vi "ZAlign.vi"(6 "Variant in":variant, 7 "Shift Pressed?":bool, 8 "error in (no error)":errorcluster, 10 "QD Combo Box Ref":refnum<vi>, 11 "QD Launch VI Ref":refnum<vi>) -> (0 "error out":errorcluster, 4 "Variant out":variant)   [LabVIEW 2014, in "ZAlign.lvlib"]
doc: "ZAlign.lvlib:ZAlign.vi\n----------------------------------------------\nQuickDrop Funktion ZAlign\n\nAuf einem Frontpanel werden alle Controls automatisch angeordnet und die Fenstergrösse eingestellt. Lokale nicht angeschlossene Controls werden unter Locals aufgeführt.\n\nTastenbefehl die ZAlign Funktion:\n1) CTRL-Space (QuickDrop starten)\n2) CTRL-A ZAlign ausführen\n\nCodebeschreibung:\n1) Das VI Fenster wird hier entsprechend der berechneten Werte eingestellt.\n2) Alle Controls erden an die neue Position verschoben.\n3) Zeichnen der Dekoartionsrahmen um die Controls\n\nDamit die Codestabilität hochgehalten werden kann, sind die VIs Passwortgeschützt. Bei Interesse und entsprechender Anfrage können die VIs aber auch entsperrt werden. \n\nInputs:\n---------------------\n- Variant in : LvVariant; \n- Shift Pressed? : Boolean; \n- error in (no error) : Cluster; \n- QD Combo Box Ref : Refnum; \n- QD Launch VI Ref : Refnum; \n\nOutputs:\n---------------------\n- error out : Cluster; \n- Variant out : LvVariant; \n\n----------------------------------------------\n16/03/2015\nZühlke Engineering AG\nCH-8952 Schlieren\nwww.zuehlke.com\n\nPLUGIN_DESCRIPTION: Zuehlke Quick Drop: ZAlign / 16.03.2015 \nPLUGIN_DEFAULT_SHORTCUT: A\n(Replace the \"$\" above with the character you wish to assign as the default shortcut for this plugin)."
uses:
  ZAlign/ZAlign.lvlib
panel:
  in  "Undo Name":string="Quick Drop Keyboard Shortcut"
  # "ZAlign!"
  # "Do not change the connector pane of this VI.\n\nSee the block diagram for directions on how to use this template."
  # "Specify the name of the Undo transaction"
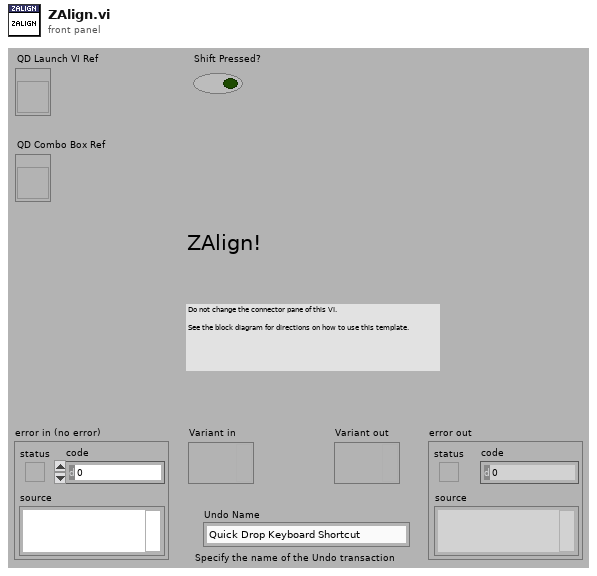
[diagram p1: front panel]
types:
  T1 = typedef "LVRectTypeDef.ctl" = cluster{"Left":i16, "Top":i16, "Right":i16, "Bottom":i16}
  T2 = cluster{"left":i16, "top":i16, "right":i16, "bottom":i16}
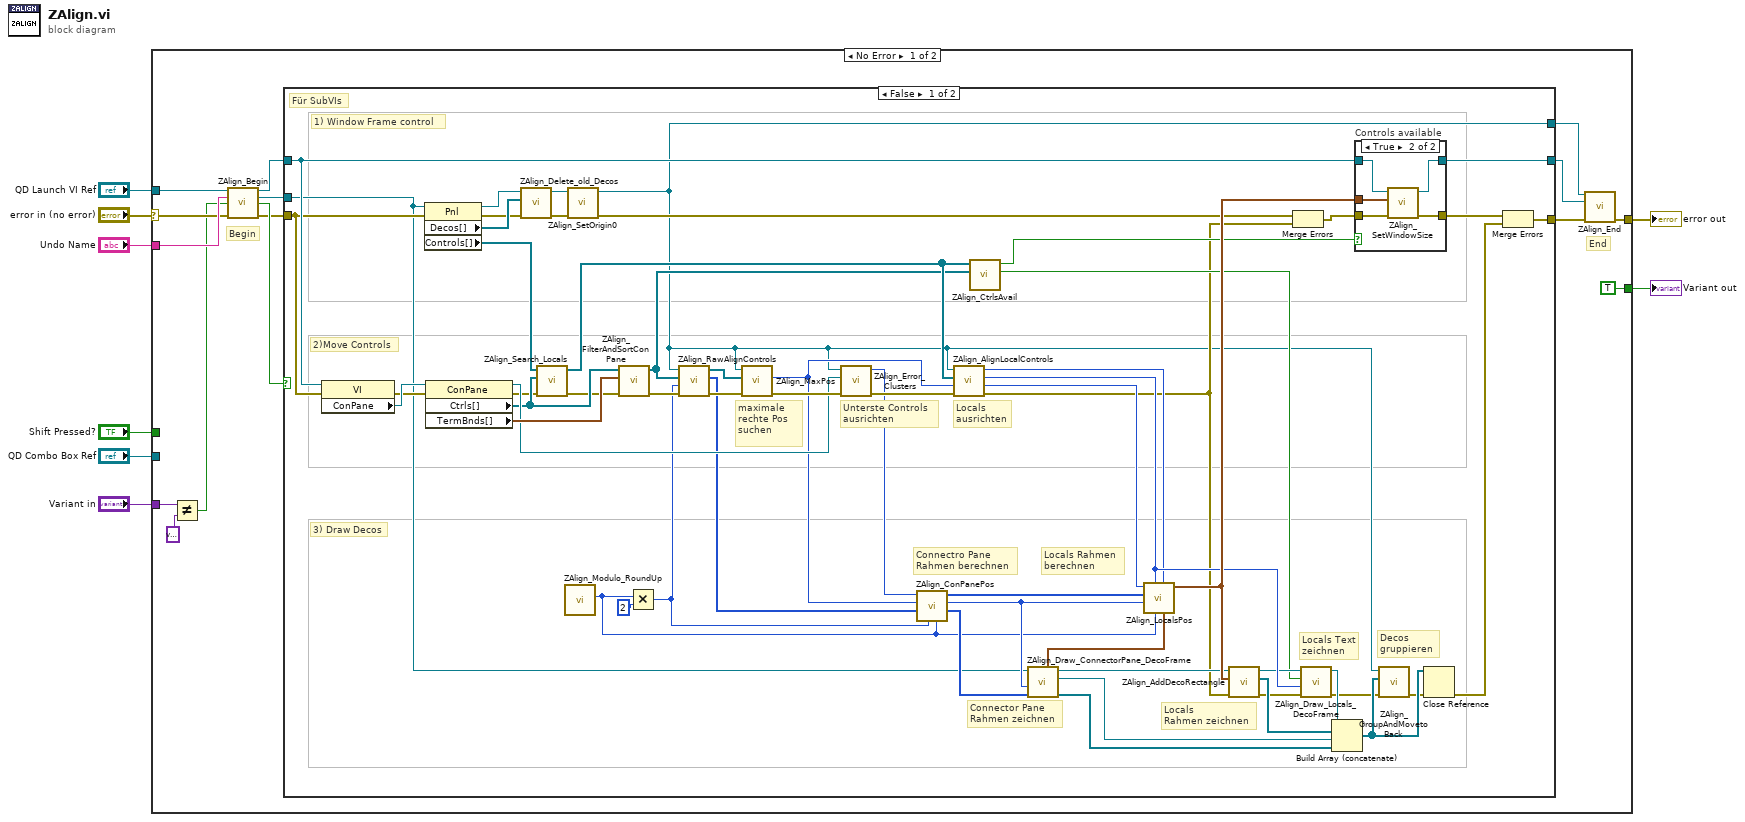
[diagram p0: block diagram]
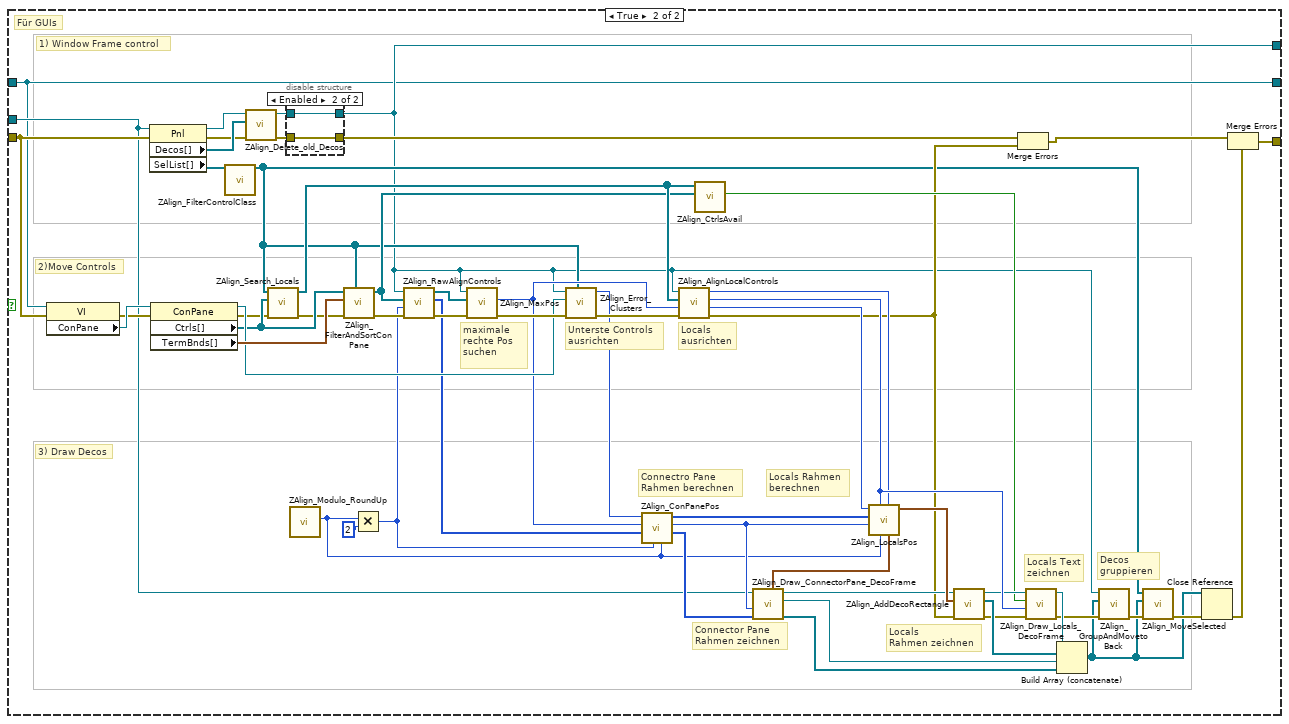
[diagram p3: hidden frame]
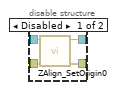
[diagram p4: hidden frame]
diagram:
  n1 = case shown="No Error" "error in (no error)" {
    selector: "error in (no error)" -> [w18 w150]
    tunnel: [w21 w150] -> w7
    tunnel: "QD Launch VI Ref" -> [w20 _]
    tunnel: "Shift Pressed?" -> [_ _]
    tunnel: "QD Combo Box Ref" -> [_ _]
    tunnel: "Variant in" -> [w11 _]
    tunnel: "Undo Name" -> [w23 _]
    tunnel: [TRUE _] -> w2
    frame No Error {
      # "End"
      # "Begin"
      n2 = Not Equal?(x=w11, y=variant) -> (x != y?=w9:bool)
      n3 = call "ZAlign_Begin.vi"("VI in"=w20, "Undo Name"=w23, "WithUndo"=w9, "error in (no error)"=w18) -> ("VIRef"=w16:refnum<vi>, "PanelRef"=w15:refnum<vi>, "SelectedElements?"=w19:bool, "error out"=w17:errorcluster)  [unwired: 8 in]
      n4 = case shown="False" w19 {
        tunnel: w17 -> [w26 w91]
        tunnel: [w65 w129] -> w14
        tunnel: w16 -> [w27 w88]
        tunnel: [w61 w88] -> w12
        tunnel: w15 -> [w25 w90]
        tunnel: [w24 w89] -> w13
        frame False {
          # "Für SubVIs"
          # "Locals Rahmen \nberechnen"
          # "Connectro Pane\nRahmen berechnen"
          # "3) Draw Decos"
          # "2)Move Controls"
          # "1) Window Frame control"
          # "Decos\ngruppieren"
          # "Locals Text\nzeichnen"
          # "Connector Pane\nRahmen zeichnen"
          # "Locals \nRahmen zeichnen"
          # "Locals\nausrichten"
          # "Unterste Controls \nausrichten"
          # "maximale\nrechte Pos\nsuchen"
          n5 = property class="VI"(reference=w27, error in=w26) -> (error out=w74:errorcluster, "ConPane"=w79:refnum<vi>)  [unwired: 1 out]
          n6 = property class="Pnl"(reference=w25, error in=w26) -> (reference out=w37:refnum<vi>, error out=w54:errorcluster, "Decos[]"=w67:refnum<vi>[], "Controls[]"=w35:refnum<vi>[])
          n7 = property class="ConPane"(reference=w79, error in=w74) -> (reference out=w75:refnum<vi>, error out=w38:errorcluster, "Ctrls[]"=w62:refnum<vi>[], "TermBnds[]"=w80:T1[])
          n8 = call "ZAlign_Delete_old_Decos.vi"("error in (no error)"=w54, "Decos[]"=w67, "Panel in"=w37) -> ("error out"=w51:errorcluster, "Panel out"=w36:refnum<vi>)  [unwired: 7 in]
          n9 = call "ZAlign_Search_Locals.vi"("error in (no error)"=w38, "Ctrls[]"=w62, "Controls[]"=w35) -> ("error out"=w52:errorcluster, "Array"=w71:refnum<vi>[])  [unwired: 7 in]
          n10 = call "ZAlign_Modulo_RoundUp.vi"() -> ("Grid_Size"=w31:i32)  [unwired: 10 in, 1 out]
          n11 = call "ZAlign_SetOrigin0.vi"("error in (no error)"=w51, "Panel in"=w36) -> ("error out"=w30:errorcluster, "reference out"=w24:refnum<vi>)  [unwired: 8 in]
          n12 = call "ZAlign_FilterAndSortConPane.vi"("error in (no error)"=w52, "TermBnds[]"=w80, "Ctrls[]"=w62) -> ("error out"=w76:errorcluster, "Ctrls[]out"=w50:refnum<vi>[])  [unwired: 7 in]
          n13 = Multiply(x=w31, y=i16 2) -> (x*y=w59:i32)
          n14 = call "ZAlign_RawAlignControls.vi"("error in (no error)"=w76, "Offset (Left and right)"=w59, "Refs"=w50, "Panel in"=w24) -> ("error out"=w77:errorcluster, "Positions"=w41:u32[], "Refs_Out"=w73:refnum<vi>[])  [unwired: 5 in]
          n15 = call "ZAlign_MaxPos.vi"("error in (no error)"=w77, "Objects"=w73, "Panel"=w24) -> ("error out"=w78:errorcluster, "Max right location"=w43:u32)  [unwired: 6 in, 1 out]
          n16 = call "ZAlign_Error_Clusters.vi"("Error in"=w78, "ConPane"=w75, "Panel"=w24) -> ("Error out"=w72:errorcluster, "Height"=w64:u32)  [unwired: 6 in, 1 out]
          n17 = call "ZAlign_ConPanePos.vi"("Grid_Size"=w31, "ScaledGridSize"=w59, "Positions"=w41, "Max right location"=w43, "Height"=w64) -> ("Positions-Grid"=w47:u32[], "Height+Grid"=w68:u32, "Positions+Grid+MaxRight"=w42:u32[])  [unwired: 4 in]
          n18 = call "ZAlign_AlignLocalControls.vi"("error in (no error)"=w72, "Max right location"=w43, "CtrlRefs"=w71, "Panel in"=w24) -> ("error out"=w28:errorcluster, "Bottom"=w40:u32, "Left"=w58:u32, "Max Right"=w44:u32)  [unwired: 4 in]
          n19 = call "ZAlign_CtrlsAvail.vi"("ConectedRefs"=w50, "LocalRefs"=w71) -> ("ConRefsAvail"=w49:bool, "RefsAvail"=w48:bool)  [unwired: 8 in]
          n20 = call "ZAlign_Draw_ConnectorPane_DecoFrame.vi"("RightPos"=w47, "Bottom"=w68, "Panel in"=w25) -> ("Deco refs"=w57:refnum<vi>[], "Decoration out"=w34:refnum<vi>, "owner refnumout"=w33:refnum<vi>, "rect"=w32:T2)  [unwired: 5 in]
          n21 = call "ZAlign_LocalsPos.vi"("rect in"=w32, "Max Right"=w44, "Grid_Size"=w31, "Left"=w58, "Height+Grid"=w68, "Positions+Grid+MaxRight"=w42, "Bottom"=w40) -> ("rect out"=w63:T2)  [unwired: 4 in]
          n22 = call "ZAlign_AddDecoRectangle.vi"("error in (no error)"=w28, "rect"=w63, "owner refnum"=w33) -> ("error out"=w53:errorcluster, "Decoration refnums"=w69:refnum<vi>[], "owner refnumout"=w56:refnum<vi>)  [unwired: 6 in]
          n23 = Merge Errors(w30, w28) -> (w29:errorcluster)
          n24 = call "ZAlign_Draw_Locals_DecoFrame.vi"("error in (no error)"=w53, "Left"=w58, "ControlsAvailable"=w49, "Generic in"=w56) -> ("error out"=w46:errorcluster, "Decoration out"=w70:refnum<vi>)  [unwired: 6 in]
          n25 = Build Array (concatenate)(w70, w69, w34, w57) -> (w66:refnum<vi>[])
          n26 = case "Controls available" shown="True" w48 {
            tunnel: w63 -> [_ w87]
            tunnel: [w81 w86] -> w61
            tunnel: [w82 w85] -> w55
            tunnel: w27 -> [w81 w84]
            tunnel: w29 -> [w82 w83]
            frame False {
            }
            frame True {
              n27 = call "ZAlign_SetWindowSize.vi"("error in (no error)"=w83, "rect"=w87, "VI in"=w84) -> ("error out"=w85:errorcluster, "reference out"=w86:refnum<vi>)  [unwired: 7 in]
            }
          }
          n28 = call "ZAlign_GroupAndMovetoBack.vi"("error in (no error)"=w46, "CtrlRefs"=w66, "Panel"=w24) -> ("error out"=w45:errorcluster)  [unwired: 8 in]
          n29 = Close Reference ("Close Ref")(reference=w66, error in (no error)=w45) -> (error out=w39:errorcluster)
          n30 = Merge Errors(w55, w39) -> (w65:errorcluster)
        }
        frame True {
          # "Für GUIs"
          # "Locals Rahmen \nberechnen"
          # "Connectro Pane\nRahmen berechnen"
          # "3) Draw Decos"
          # "2)Move Controls"
          # "1) Window Frame control"
          # "Decos\ngruppieren"
          # "Locals Text\nzeichnen"
          # "Connector Pane\nRahmen zeichnen"
          # "Locals \nRahmen zeichnen"
          # "Locals\nausrichten"
          # "Unterste Controls \nausrichten"
          # "maximale\nrechte Pos\nsuchen"
          n31 = property class="VI"(reference=w88, error in=w91) -> (error out=w137:errorcluster, "ConPane"=w142:refnum<vi>)  [unwired: 1 out]
          n32 = property class="Pnl"(reference=w90, error in=w91) -> (reference out=w107:refnum<vi>, error out=w121:errorcluster, "Decos[]"=w130:refnum<vi>[], "SelList[]"=w101:refnum<vi>[])
          n33 = property class="ConPane"(reference=w142, error in=w137) -> (reference out=w138:refnum<vi>, error out=w108:errorcluster, "Ctrls[]"=w126:refnum<vi>[], "TermBnds[]"=w143:T1[])
          n34 = call "ZAlign_FilterControlClass.vi"("SelList[]"=w101) -> ("CtrlRefArray"=w92:refnum<vi>[])  [unwired: 14 in]
          n35 = call "ZAlign_Delete_old_Decos.vi"("error in (no error)"=w121, "Decos[]"=w130, "Panel in"=w107) -> ("error out"=w94:errorcluster, "Panel out"=w95:refnum<vi>)  [unwired: 7 in]
          n36 = call "ZAlign_Search_Locals.vi"("error in (no error)"=w108, "Ctrls[]"=w126, "Controls[]"=w92) -> ("error out"=w119:errorcluster, "Array"=w134:refnum<vi>[])  [unwired: 7 in]
          n37 = disable-structure shown="Enabled" {
            disable-tunnel: w95 -> [w147 w149]
            disable-tunnel: [w146 w149] -> w89
            disable-tunnel: w94 -> [w145 w148]
            disable-tunnel: [w144 w148] -> w93
            frame Disabled {
              n38 = call "ZAlign_SetOrigin0.vi"("error in (no error)"=w145, "Panel in"=w147) -> ("error out"=w144:errorcluster, "reference out"=w146:refnum<vi>)  [unwired: 8 in]
            }
            frame Enabled {
            }
          }
          n39 = call "ZAlign_Modulo_RoundUp.vi"() -> ("Grid_Size"=w103:i32)  [unwired: 10 in, 1 out]
          n40 = call "ZAlign_FilterAndSortConPane.vi"("FilterCtrls[]"=w92, "error in (no error)"=w119, "TermBnds[]"=w143, "Ctrls[]"=w126) -> ("error out"=w139:errorcluster, "Ctrls[]out"=w118:refnum<vi>[])  [unwired: 6 in]
          n41 = Multiply(x=w103, y=i16 2) -> (x*y=w99:i32)
          n42 = call "ZAlign_RawAlignControls.vi"("error in (no error)"=w139, "Offset (Left and right)"=w99, "Refs"=w118, "Panel in"=w89) -> ("error out"=w140:errorcluster, "Positions"=w111:u32[], "Refs_Out"=w136:refnum<vi>[])  [unwired: 5 in]
          n43 = call "ZAlign_MaxPos.vi"("error in (no error)"=w140, "Objects"=w136, "Panel"=w89) -> ("error out"=w141:errorcluster, "Max right location"=w113:u32)  [unwired: 6 in, 1 out]
          n44 = call "ZAlign_Error_Clusters.vi"("FilterCtrls[]"=w92, "Error in"=w141, "ConPane"=w138, "Panel"=w89) -> ("Error out"=w135:errorcluster, "Height"=w128:u32)  [unwired: 5 in, 1 out]
          n45 = call "ZAlign_ConPanePos.vi"("Grid_Size"=w103, "ScaledGridSize"=w99, "Positions"=w111, "Max right location"=w113, "Height"=w128) -> ("Positions-Grid"=w116:u32[], "Height+Grid"=w131:u32, "Positions+Grid+MaxRight"=w112:u32[])  [unwired: 4 in]
          n46 = call "ZAlign_AlignLocalControls.vi"("error in (no error)"=w135, "Max right location"=w113, "CtrlRefs"=w134, "Panel in"=w89) -> ("error out"=w102:errorcluster, "Bottom"=w110:u32, "Left"=w124:u32, "Max Right"=w114:u32)  [unwired: 4 in]
          n47 = call "ZAlign_CtrlsAvail.vi"("ConectedRefs"=w118, "LocalRefs"=w134) -> ("ConRefsAvail"=w117:bool)  [unwired: 8 in, 1 out]
          n48 = call "ZAlign_Draw_ConnectorPane_DecoFrame.vi"("RightPos"=w116, "Bottom"=w131, "Panel in"=w90) -> ("Deco refs"=w123:refnum<vi>[], "Decoration out"=w106:refnum<vi>, "owner refnumout"=w105:refnum<vi>, "rect"=w104:T2)  [unwired: 5 in]
          n49 = call "ZAlign_LocalsPos.vi"("rect in"=w104, "Max Right"=w114, "Grid_Size"=w103, "Left"=w124, "Height+Grid"=w131, "Positions+Grid+MaxRight"=w112, "Bottom"=w110) -> ("rect out"=w127:T2)  [unwired: 4 in]
          n50 = call "ZAlign_AddDecoRectangle.vi"("error in (no error)"=w102, "rect"=w127, "owner refnum"=w105) -> ("error out"=w120:errorcluster, "Decoration refnums"=w132:refnum<vi>[], "owner refnumout"=w122:refnum<vi>)  [unwired: 6 in]
          n51 = Merge Errors(w93, w102) -> (w100:errorcluster)
          n52 = call "ZAlign_Draw_Locals_DecoFrame.vi"("error in (no error)"=w120, "Left"=w124, "ControlsAvailable"=w117, "Generic in"=w122) -> ("error out"=w115:errorcluster, "Decoration out"=w133:refnum<vi>)  [unwired: 6 in]
          n53 = Build Array (concatenate)(w133, w132, w106, w123) -> (w96:refnum<vi>[])
          n54 = call "ZAlign_GroupAndMovetoBack.vi"("error in (no error)"=w115, "CtrlRefs"=w96, "Panel"=w89) -> ("error out"=w98:errorcluster)  [unwired: 8 in]
          n55 = call "ZAlign_MoveSelected.vi"("error in (no error)"=w98, "CtrlRefs"=w96, "Controls"=w92) -> ("error out"=w97:errorcluster)  [unwired: 8 in]
          n56 = Close Reference ("Close Ref")(reference=w96, error in (no error)=w97) -> (error out=w109:errorcluster)
          n57 = Merge Errors(w100, w109) -> (w129:errorcluster)
        }
      }
      n58 = call "ZAlign_End.vi"("Panel in"=w13, "VI in"=w12, "error in (no error)"=w14) -> ("error out"=w21:errorcluster)  [unwired: 12 in]
    }
    frame Error {
    }
  }
  "error out" <- w7
  "Variant out" <- w2
